vi "DAQmx Create Channel (AI-Force-Bridge-Table).vi"(0 "task in":refnum<k21>, 1 "maximum value":dbl=100.0 format="%0.2f", 2 "minimum value":dbl=-100.0 format="%0.2f", 3 "bridge information":T1={"bridge configuration"=10182, "voltage excitation source"=10200, "voltage excitation value"=2.5, "nominal bridge resistance"=350.0} {"voltage excitation source" items=["Internal"=10200, "External"=10167]; "bridge configuration" items=["Full Bridge"=10182, "Half Bridge"=10187, "Quarter Bridge"=10270]}, 5 "physical channels":tag, 7 "name to assign":string, 9 "units":i32(ring)=15876 items=["Newtons"=15875, "Pounds"=15876, "kgf"=15877, "From Custom Scale"=10065], 11 "error in":errorcluster, 12 "custom scale name":tag, 14 "scaling information":T2={"electrical values"=[-2.0, 0.0, 2.0], "electrical units"=15897, "physical values"=[-100.0, 0.0, 100.0], "physical units"=15876} {"physical units" items=["Newtons"=15875, "Pounds"=15876, "kgf"=15877]; "electrical units" items=["Volts/Volt"=15896, "mVolts/Volt"=15897]}) -> (4 "task out":refnum<k21>, 15 "error out":errorcluster)   [LabVIEW 2018]
doc: "Creates channel(s) that use a Wheatstone bridge to measure force or load. Use this instance with sensors whose specifications provide a table of electrical values and the corresponding physical values. When you use this scaling type, NI-DAQmx performs linear scaling between each pair of electrical and physical values. The input limits specified with <B>minimum value</B> and <B>maximum value</B> must fall within the smallest and largest physical values. For any data outside those endpoints, NI-DAQmx coerces that data to the endpoints."
uses:
  nilvaiu.dll
panel:
  # "input limits"
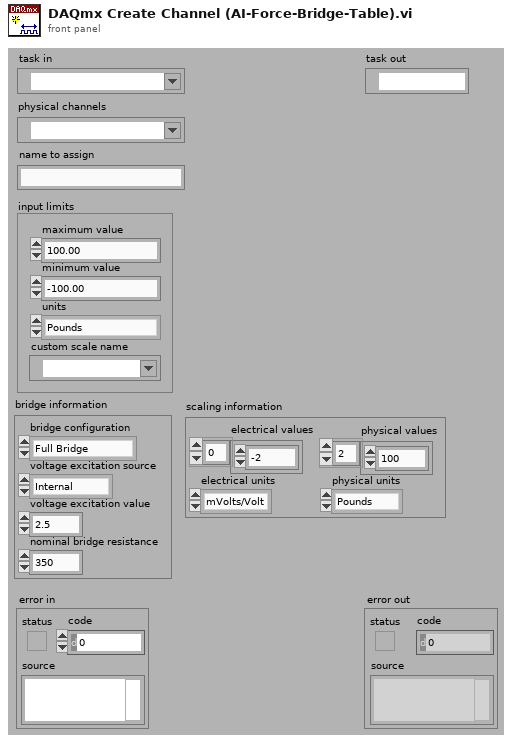
[diagram p1: front panel]
types:
  T1 = cluster{"bridge configuration":i32, "voltage excitation source":i32, "voltage excitation value":dbl, "nominal bridge resistance":dbl}
  T2 = cluster{"electrical values":dbl[], "electrical units":i32, "physical values":dbl[], "physical units":i32}
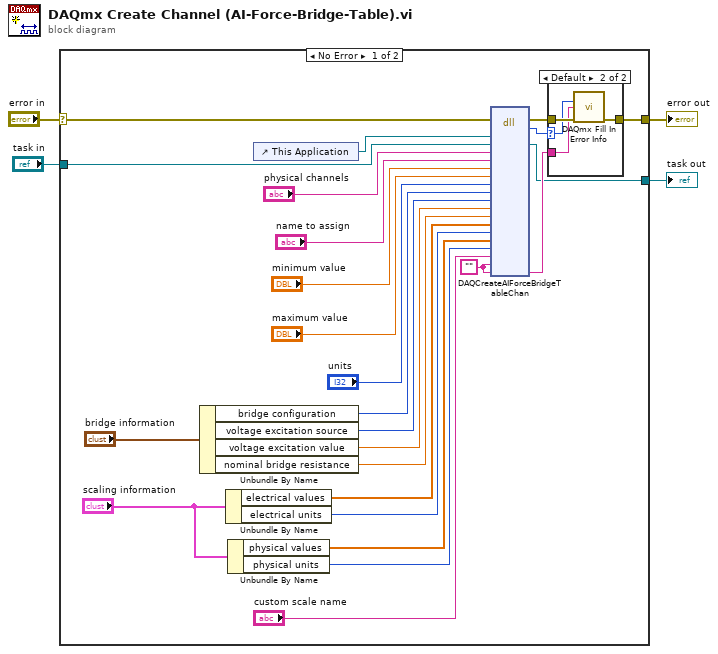
[diagram p0: block diagram]
diagram:
  n1 = case shown="No Error" "error in" {
    selector: "error in" -> [w25 w35]
    tunnel: [w10 w35] -> w4
    tunnel: "task in" -> [w7 w36]
    tunnel: [w8 w36] -> w1
    frame No Error {
      w5 = ""
      n2 = Unbundle By Name("bridge information") -> ("bridge configuration"=w16:i32, "voltage excitation source"=w15:i32, "voltage excitation value"=w14:dbl, "nominal bridge resistance"=w13:dbl)
      n3 = Unbundle By Name("scaling information") -> ("electrical values"=w20:dbl[], "electrical units"=w19:i32)
      n4 = Unbundle By Name("scaling information") -> ("physical values"=w18:dbl[], "physical units"=w17:i32)
      n5 = control-ref of="This Application"() -> (w27:refnum<vi>)
      n6 = dll-call lib="nilvaiu.*" fn="DAQCreateAIForceBridgeTableChan"(error in=w25, "lvAppRef"=w27, "refObjPtr"=w7, "physicalChannelName"="physical channels", "channelNameIn"="name to assign", "minVal"="minimum value", "maxVal"="maximum value", "units"="units", "bridgeConfig"=w16, "voltageExcitSource"=w15, "voltageExcitVal"=w14, "nominalBridgeResistance"=w13, "electricalValues"=w20, "electricalUnits"=w19, "physicalValues"=w18, "physicalUnits"=w17, "customScaleName"="custom scale name", "channelNamesOut"=w5, "extendedErrorInfo"=w5) -> (error out=w11:errorcluster, "return type"=w9:i32, "refObjPtr"=w8:refnum<k21>, "extendedErrorInfo"=w12:string)  [unwired: 18 in, 1 out]
      n7 = case shown="Default" w9 {
        selector: w9 -> [_ w32]
        tunnel: w11 -> [w30 w34]
        tunnel: [w30 w33] -> w10
        tunnel: w12 -> [_ w31]
        frame 0 {
        }
        frame Default {
          n8 = call "DAQmx Fill In Error Info.vi"("status code"=w32, "extended error info"=w31, "error in"=w34) -> ("error out"=w33:errorcluster)  [unwired: 1 in, 11 out]
        }
      }
    }
    frame Error {
    }
  }
  "error out" <- w4
  "task out" <- w1
